vi "Chart-Get Overview Limit.vi"(8 "error in":errorcluster, 11 "Overview Refnum In":refnum<vi>) -> (0 "error out":errorcluster, 2 "Limit":cluster{"Lower Limit":dbl, "Upper Limit":dbl}, 3 "Overview Refnum Out":refnum<vi>)   [LabVIEW 2020]
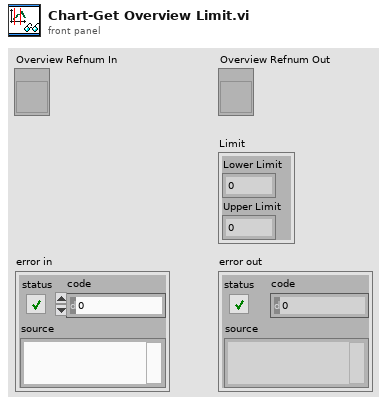
[diagram p1: front panel]
types:
  T1 = cluster{"Cursor.Cursor X":dbl, "Cursor.Cursor X":dbl}
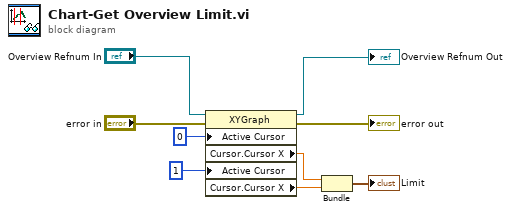
[diagram p0: block diagram]
diagram:
  n1 = property class="XYGraph"(reference="Overview Refnum In", error in="error in", "Active Cursor"=u32 0, "Active Cursor"=u32 1) -> (reference out=→"Overview Refnum Out":refnum<vi>, error out=→"error out":errorcluster, "Cursor.Cursor X"=w2:dbl, "Cursor.Cursor X"=w3:dbl)
  n2 = Bundle("Cursor.Cursor X"=w2, "Cursor.Cursor X"=w3) -> (→"Limit":T1)  [unwired: 1 in]
